vi "GetNetworkTime.vi"(8 "error in (no error)":errorcluster, 11 "NetworkImpairmentPluginBase in":refnum<class "NetworkImpairmentPluginBase.lvclass">) -> (0 "error out":errorcluster, 3 "NetworkImpairmentPluginBase out":refnum<class "NetworkImpairmentPluginBase.lvclass">)   [LabVIEW 2014, in "NetworkImpairmentPlugins.lvlib" / "NetworkImpairmentPluginBase.lvclass"]
uses:
  NetworkImpairmentPluginBase.lvclass
  <userlib>/NIST/BaseClasses/Object_class/BaseObject.lvclass
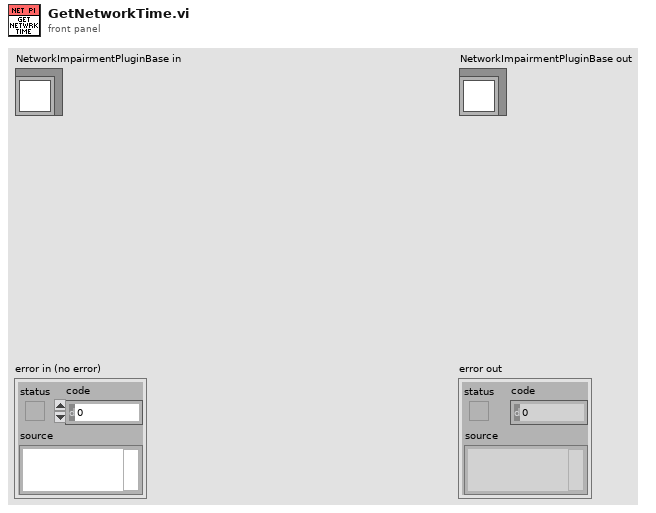
[diagram p1: front panel]
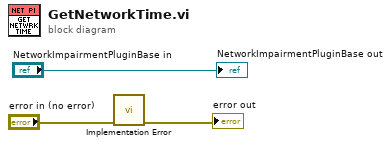
[diagram p0: block diagram]
diagram:
  n1 = call <userlib>:"Implementation Error.vi"("error in (no error)"="error in (no error)") -> ("error out"=→"error out":errorcluster)  [unwired: 10 in]
  "NetworkImpairmentPluginBase out" <- "NetworkImpairmentPluginBase in"
